vi "Define_Indicies_of_Earliest_Pr_Dot-1.vi"(4 "error IN":errorcluster, 6 "[IN] #of Frames":i32, 7 "[IN] Still connected\ntracks in group":T1) -> (0 "error OUT":errorcluster, 2 "[OUT] Index of Subtrack":i32, 3 "[OUT] Index of Ear\nliest Problem Point":i32)   [LabVIEW 2017]
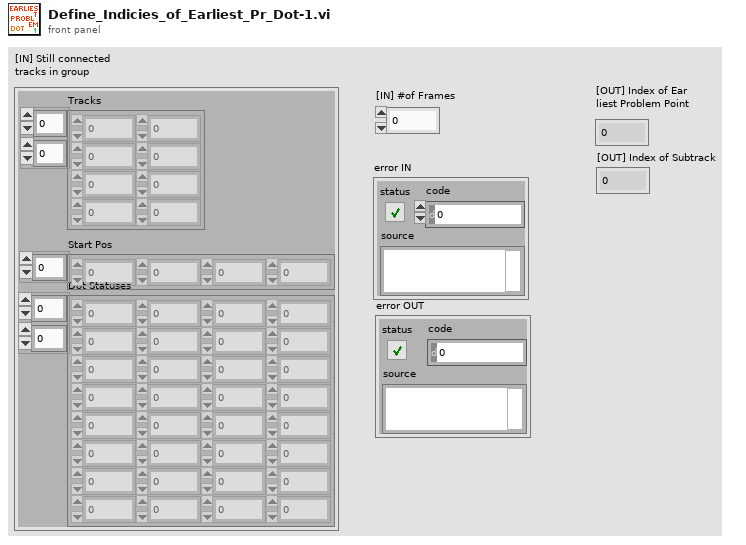
[diagram p1: front panel]
types:
  T1 = cluster{"Tracks":dbl[][], "Start Pos":i32[], "Dot Statuses":i16[][]}
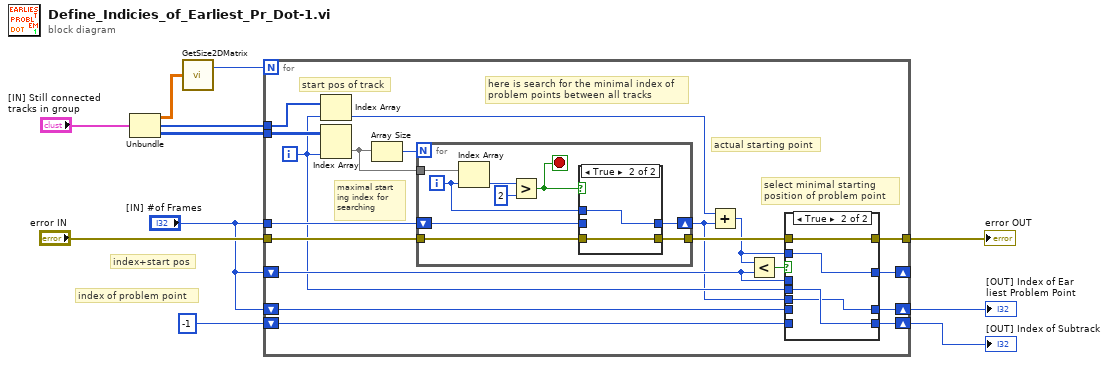
[diagram p0: block diagram]
diagram:
  # "index of problem point"
  # "index+start pos"
  n1 = Unbundle("[IN] Still connected\ntracks in group") -> ("Tracks"=w11:dbl[][], "Start Pos"=w10:i32[], "Dot Statuses"=w6:i16[][])
  n2 = call "GetSize2DMatrix.vi"("Array IN (2D)"=w11) -> ("# Cols"=w9:i32)  [unwired: 1 out]
  n3 = for {
    N: w9 -> [_]
    tunnel: w6 -> [w30]
    tunnel: w10 -> [w29]
    shift-right: [w23] -> _
    shift-left: "[IN] #of Frames" -> [w24]
    tunnel: "[IN] #of Frames" -> [w26]
    tunnel: "error IN" -> [w22]
    tunnel: [w20] -> w2
    shift-right: [w17] -> w1
    shift-left: -1 ("# Cols") -> [w19]
    shift-right: [w13] -> w3
    shift-left: "[IN] #of Frames" -> [w14]
    i -> [w18]
    # "actual starting point"
    # "here is search for the minimal index of \nproblem points between all tracks"
    # "select minimal starting \nposition of problem point"
    # "maximal start\ning index for\nsearching"
    # "start pos of track"
    n4 = Index Array(array=w29, index=w18) -> (element=w16:i32)
    n5 = Index Array(array=w30, index (col)=w18) -> (element=w27:i16[])  [unwired: 1 in]
    n6 = Array Size(array=w27) -> (size(s)=w28:i32)
    n7 = for {
      N: w28 -> [_]
      tunnel: w27 -> [w47]
      shift-right: [w41] -> w12
      shift-left: w26 -> [w43]
      tunnel: w22 -> [w40]
      tunnel: [w39] -> w21
      i -> [w42]
      stop <- w44 stop-if-true
      n8 = Index Array(array=w47, index=w42) -> (element=w46:i16)
      n9 = Greater?(x=w46, y=i16 2) -> (0:w44:bool)
      n10 = case shown="True" w44 {
        tunnel: w43 -> [w49 _]
        tunnel: w42 -> [_ w51]
        tunnel: [w49 w51] -> w41
        tunnel: w40 -> [w48 w50]
        tunnel: [w48 w50] -> w39
        frame False {
        }
        frame True {
        }
      }
    }
    n11 = Add(x=w16, y=w12) -> (x+y=w15:i32)
    n12 = Less?(x=w15, y=w24) -> (x < y?=w25:bool)
    n13 = case shown="True" w25 {
      tunnel: w24 -> [w34 _]
      tunnel: [w34 w38] -> w23
      tunnel: w15 -> [_ w38]
      tunnel: w21 -> [w33 w37]
      tunnel: [w33 w37] -> w20
      tunnel: w19 -> [w32 _]
      tunnel: w18 -> [_ w36]
      tunnel: [w32 w36] -> w17
      tunnel: w14 -> [w31 _]
      tunnel: [w31 w35] -> w13
      tunnel: w12 -> [_ w35]
      frame False {
        # "index"
        # "index+start\npos"
      }
      frame True {
      }
    }
  }
  "[OUT] Index of Ear\nliest Problem Point" <- w3
  "error OUT" <- w2
  "[OUT] Index of Subtrack" <- w1
